vi "Running Avg.vi"(6 "Window Width (ds)":dbl format="%#_13g", 8 "error in":errorcluster, 9 "mode":bool, 10 "Samples cnt":i32, 11 "Data In":dbl[](array[numeric])) -> (0 "error out":errorcluster, 2 "Corrected":dbl[](array[numeric]), 3 "Avg out":dbl[](array[numeric]))   [LabVIEW 2019]
uses:
  <vilib>/Analysis/NI_AALBase.lvlib
panel:
  out "Variance":dbl[](array[numeric])
  out "Écart Type":dbl[](array[numeric])
  out "Averaging groups":dbl[][](array[numeric])
  out "Graphe":dbl[][](graph)
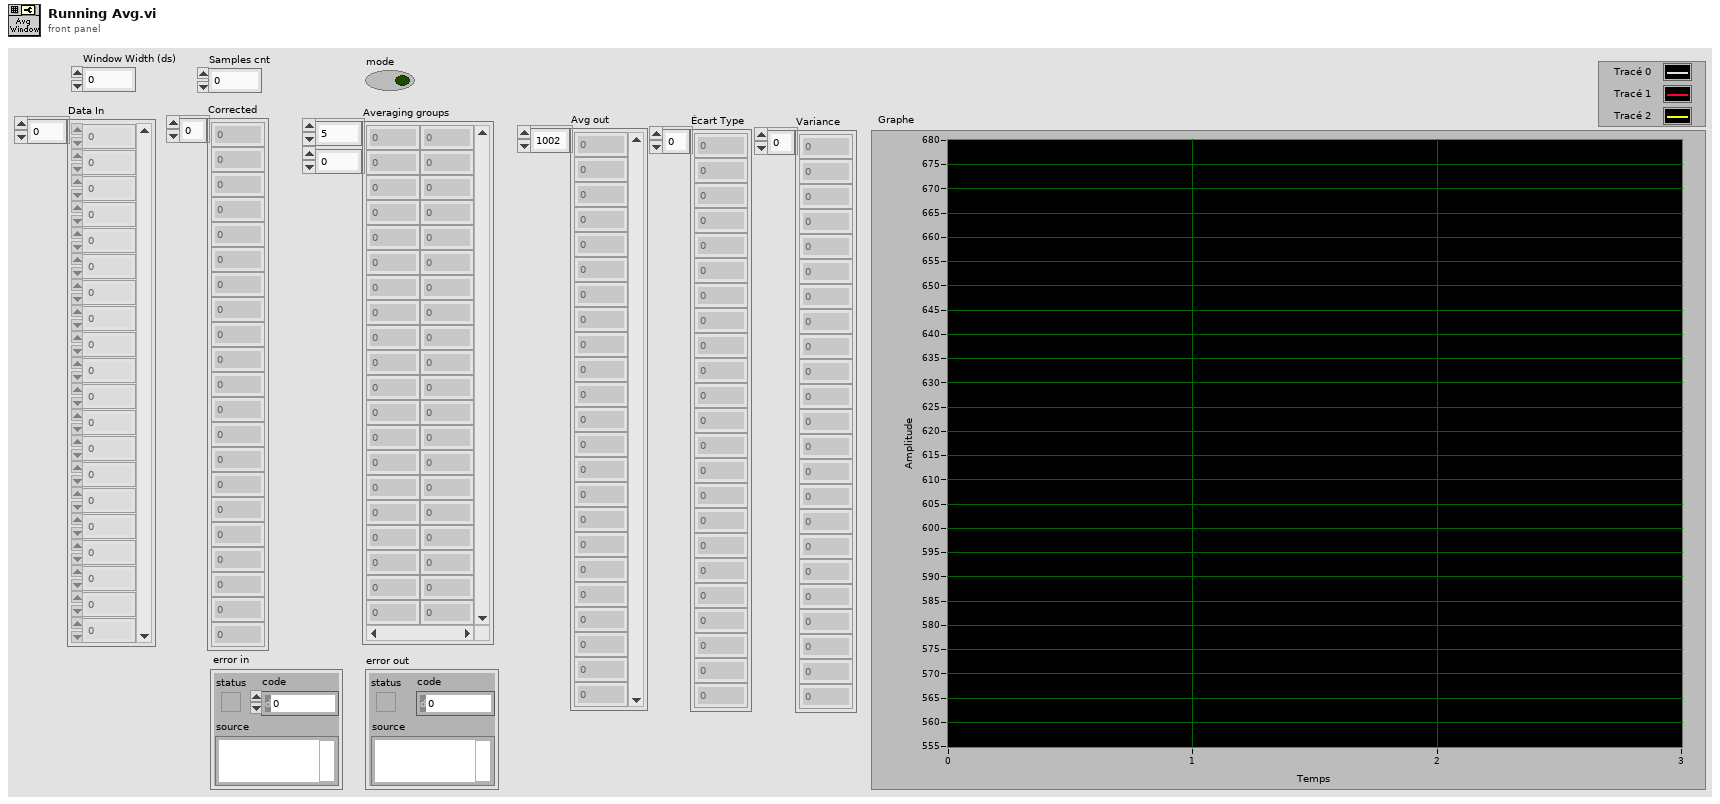
[diagram p1: front panel]
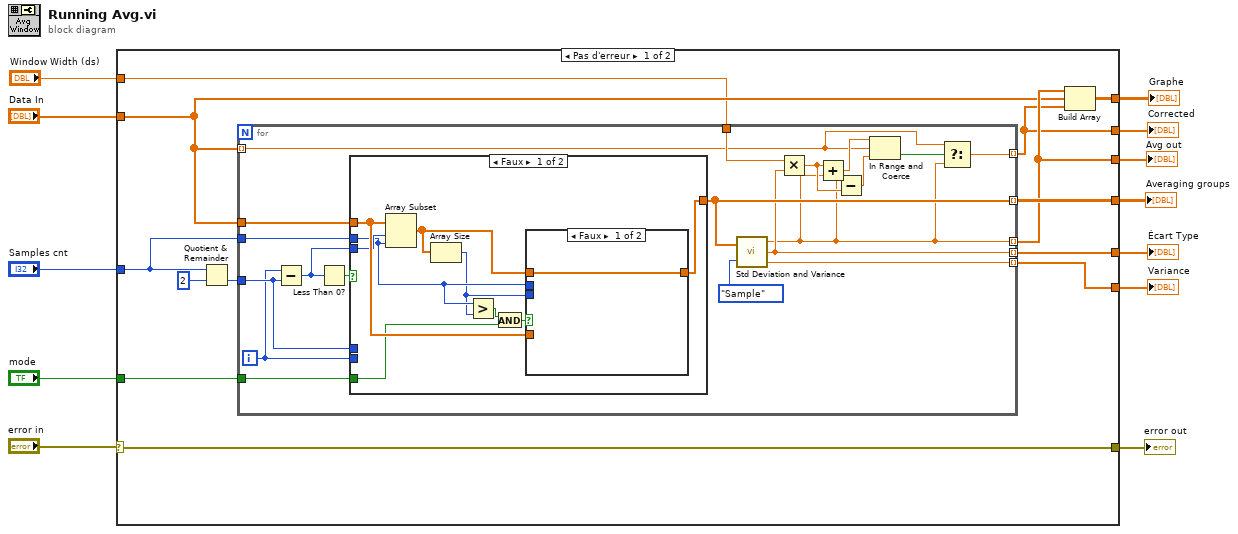
[diagram p0: block diagram]
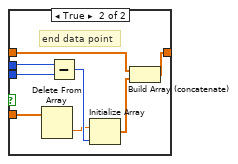
[diagram p2: hidden frame]
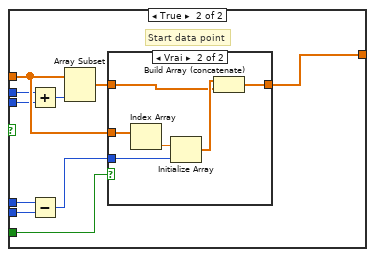
[diagram p3: hidden frame]
diagram:
  n1 = case shown="Pas d'erreur" "error in" {
    selector: "error in" -> [w16 w80]
    tunnel: "Samples cnt" -> [w24 _]
    tunnel: "mode" -> [w22 _]
    tunnel: [w21 _] -> w10
    tunnel: [w20 _] -> w9
    tunnel: "Data In" -> [w15 _]
    tunnel: [w19 _] -> w7
    tunnel: [w18 _] -> w6
    tunnel: [w17 _] -> w5
    tunnel: [w16 w80] -> w3
    tunnel: "Window Width (ds)" -> [w14 _]
    tunnel: [w13 _] -> w1
    frame No Error {
      n2 = Quotient & Remainder(x=w24, y=2) -> (floor(x/y)=w23:i32)  [unwired: 1 out]
      n3 = for {
        tunnel: w15 -> [w44]
        tunnel: w24 -> [w43]
        tunnel: w23 -> [w40]
        tunnel: [w28] -> w19 mode=indexing
        tunnel: w22 -> [w39]
        tunnel: [w37] -> w21 mode=indexing
        tunnel: [w34] -> w18 mode=indexing
        tunnel: [w35] -> w17 mode=indexing
        tunnel: w14 -> [w33]
        tunnel: w15 -> [w29] mode=indexing
        tunnel: [w26] -> w13 mode=indexing
        i -> [w38]
        n4 = Subtract(x=w38, y=w40) -> (x-y=w42:i32)
        n5 = Less Than 0?(x=w42) -> (x < 0?=w41:bool)
        n6 = case shown="Faux" w41 {
          tunnel: w44 -> [w53 w72]
          tunnel: w42 -> [w52 w69]
          tunnel: w43 -> [w51 w68]
          tunnel: w40 -> [_ w71]
          tunnel: w39 -> [w45 w63]
          tunnel: [w46 w64] -> w37
          tunnel: w38 -> [_ w65]
          frame False {
            n7 = Array Subset(array=w53, index=w52, length=w51) -> (w47:dbl[])
            n8 = Array Size(array=w47) -> (size(s)=w50:i32)
            n9 = Greater?(x=w51, y=w50) -> (0:w49:bool)
            n10 = And(x=w49, y=w45) -> (x .and. y?=w48:bool)
            n11 = case shown="Faux" w48 {
              tunnel: w53 -> [_ w56]
              tunnel: w51 -> [_ w62]
              tunnel: w50 -> [_ w61]
              tunnel: w47 -> [w54 w58]
              tunnel: [w54 w57] -> w46
              frame False {
              }
              frame True {
                # "end data point"
                n12 = Delete From Array(array=w56) -> (deleted portion=w55:dbl)  [unwired: 2 in, 1 out]
                n13 = Subtract(x=w62, y=w61) -> (x-y=w60:i32)
                n14 = Initialize Array(w55, w60) -> (w59:dbl[])
                n15 = Build Array (concatenate)(w58, w59) -> (w57:dbl[])
              }
            }
          }
          frame True {
            # "Start data point"
            n16 = Add(x=w68, y=w69) -> (x+y=w67:i32)
            n17 = Subtract(x=w71, y=w65) -> (x-y=w66:i32)
            n18 = Array Subset(array=w72, length=w67) -> (w70:dbl[])  [unwired: 1 in]
            n19 = case shown="Vrai" w63 {
              tunnel: w72 -> [_ w79]
              tunnel: w66 -> [_ w77]
              tunnel: w70 -> [w73 w75]
              tunnel: [w73 w74] -> w64
              frame False {
              }
              frame True {
                n20 = Index Array(array=w79) -> (element=w78:dbl)  [unwired: 1 in]
                n21 = Initialize Array(w78, w77) -> (w76:dbl[])
                n22 = Build Array (concatenate)(w76, w75) -> (w74:dbl[])
              }
            }
          }
        }
        n23 = call <vilib>:"Std Deviation and Variance.vi"("X"=w37, "Weighting (Sample)"=enum16{"Sample", "Population"}."Sample") -> ("mean"=w28:dbl, "standard deviation"=w34:dbl, "variance"=w35:dbl)
        n24 = Multiply(x=w33, y=w34) -> (x*y=w31:dbl)
        n25 = Add(x=w31, y=w28) -> (x+y=w32:dbl)
        n26 = Subtract(x=w28, y=w31) -> (x-y=w30:dbl)
        n27 = In Range and Coerce(upper limit=w32, x=w29, lower limit=w30) -> (In Range?=w27:bool)  [unwired: 1 out]
        n28 = Select(t=w29, s=w27, f=w28) -> (s? t:f=w26:dbl)
      }
      n29 = Build Array(w19, w15, w13) -> (w20:dbl[][])
    }
    frame Error {
    }
  }
  "Graphe" <- w9
  "Avg out" <- w7
  "Averaging groups" <- w10
  "error out" <- w3
  "Écart Type" <- w6
  "Variance" <- w5
  "Corrected" <- w1
